vi "Begin.vi"(11 "Image Size":T1=enum."160x120") -> (0 "error out":errorcluster)   [LabVIEW 2013]
doc: "Called before other user functions, this VI is expected to open initial I/O refnums, load in file data, and do all program initialization. Notice that the <B>error out</B> terminal is simply used for data flow. Wiring it to other structures or subVIs ensures that this VI runs first."
uses:
  <vilib>/Rock Robotics/WPI/Camera/WPI_CameraImageSize.ctl
  <vilib>/Rock Robotics/SystemInterfaces/DIO/FPGA_DIOPWMChannel.ctl
  <vilib>/Rock Robotics/WPI/Camera/WPI_CameraWhite Balance Values.ctl
  <vilib>/Rock Robotics/WPI/Camera/WPI_CameraExposure Values.ctl
  <vilib>/Rock Robotics/WPI/Camera/WPI_CameraFrameRate.ctl
  <vilib>/Rock Robotics/WPI/DriverStation/WPI_DriverStationRobotMode2.ctl
  <vilib>/Rock Robotics/WPI/Joystick/WPI_JoystickDeviceEnum.ctl
  <vilib>/Rock Robotics/WPI/Solenoid/WPI_SolenoidChannel.ctl
  <vilib>/Rock Robotics/SystemInterfaces/DIO/FPGA_DIOChannel.ctl
  <vilib>/Rock Robotics/SystemInterfaces/DIO/FPGA_DIORelayChannel.ctl
  <vilib>/Rock Robotics/WPI/SafetyOutput/WPI_SafetyOutputConfigMenu.ctl
  <vilib>/Rock Robotics/SystemInterfaces/AI/FPGA_AIChannel.ctl
  <vilib>/Rock Robotics/SystemInterfaces/Typedef/FPGA_TypedefAnalogModule.ctl
  <vilib>/Rock Robotics/SystemInterfaces/AI/FPGA_AIGyroChannel.ctl
  <vilib>/Rock Robotics/SystemInterfaces/Typedef/FPGA_TypedefAnalogModuleForGyro.ctl
  <vilib>/Rock Robotics/SystemInterfaces/Typedef/FPGA_TypedefDigitalModule.ctl
  <vilib>/Rock Robotics/WPI/RobotDrive/WPI_RobotDriveOpen2MotorWithTalon.vi
  Robot Global Data.vi
  <vilib>/Rock Robotics/WPI/Solenoid/WPI_SolenoidOpenSingle.vi
  <vilib>/Rock Robotics/WPI/MotorControl/WPI_MotorControlOpen Victor.vi
  <vilib>/Rock Robotics/WPI/Counter/WPI_CounterDigitalInputToDigitalSource.vi
  <vilib>/Rock Robotics/WPI/Counter/WPI_CounterOpen Gear Tooth Sensor Mode.vi
  <vilib>/Rock Robotics/WPI/Compressor/WPI_CompressorGetSetRefNum.vi
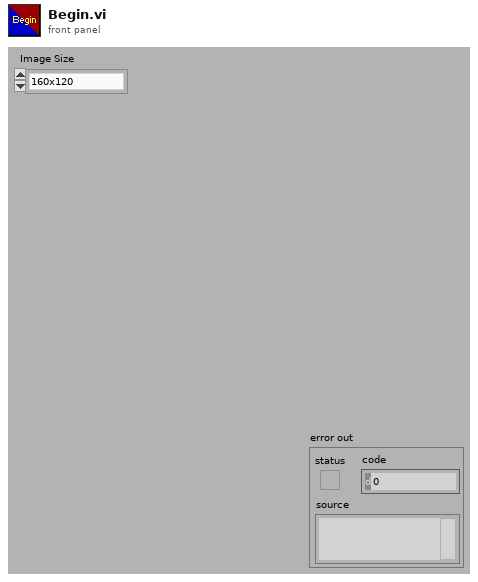
[diagram p1: front panel]
types:
  T1 = typedef "WPI_CameraImageSize.ctl" = enum16{"640x480", "320x240", "160x120"}
  T2 = typedef "WPI_SolenoidChannel.ctl" = enum8{"Solenoid 1", "Solenoid 2", "Solenoid 3", "Solenoid 4", "Solenoid 5", "Solenoid 6", "Solenoid 7", "Solenoid 8", "Invalid"}
  T3 = typedef "FPGA_TypedefDigitalModule.ctl" = enum16{"Digital Module 1", "Digital Module 2"}
  T4 = typedef "FPGA_DIOChannel.ctl" = enum8{"DIO 1", "DIO 2", "DIO 3", "DIO 4", "DIO 5", "DIO 6", "DIO 7", "DIO 8", "DIO 9", "DIO 10", "DIO 11", "DIO 12", "DIO 13", "DIO 14", "Invalid"}
  T5 = typedef "FPGA_TypedefAnalogModuleForGyro.ctl" = enum16{"Analog Module 1"}
  T6 = typedef "FPGA_AIGyroChannel.ctl" = enum8{"AI 1", "AI 2", "Invalid"}
  T7 = typedef "WPI_JoystickDeviceEnum.ctl" = enum16{"USB 1", "USB 2", "USB 3", "USB 4", "Kinect 1", "Kinect 2"}
  T8 = typedef "FPGA_TypedefAnalogModule.ctl" = enum16{"Analog Module 1", "Analog Module 2"}
  T9 = typedef "FPGA_AIChannel.ctl" = enum8{"AI 1", "AI 2", "AI 3", "AI 4", "AI 5", "AI 6", "AI 7", "AI 8", "Invalid"}
  T10 = typedef "WPI_SafetyOutputConfigMenu.ctl" = enum16{"Enable", "Disable"}
  T11 = typedef "FPGA_DIORelayChannel.ctl" = enum8{"Relay 1", "Relay 2", "Relay 3", "Relay 4", "Relay 5", "Relay 6", "Relay 7", "Relay 8", "Invalid"}
  T12 = typedef "FPGA_DIOPWMChannel.ctl" = enum8{"PWM 1", "PWM 2", "PWM 3", "PWM 4", "PWM 5", "PWM 6", "PWM 7", "PWM 8", "PWM 9", "PWM 10", "Invalid"}
  T13 = typedef "WPI_DriverStationRobotMode2.ctl" = enum16{"Autonomous Disabled", "Autonomous Enabled", "Teleop Disabled", "Teleop Enabled", "Timeout", "Finish", "Test Disabled", "Test Enabled"}
  T14 = typedef "WPI_CameraFrameRate.ctl" = u32
  T15 = typedef "WPI_CameraExposure Values.ctl" = enum16{"Auto", "Flicker-free 50 Hz", "Flicker-free 60 Hz", "Hold current"}
  T16 = typedef "WPI_CameraWhite Balance Values.ctl" = enum16{"Auto", "Fixed indoor", "Fixed outdoor 1", "Fixed outdoor 2", "Fixed fluorescent 1", "Fixed fluorescent 2", "Hold current"}
  T17 = typedef "WPI_SolenoidDevRef.ctl" = cluster{"DevStatus":errorcluster, "Solenoid Module":T18, "Forward Solenoid Channel":T2, "Reverse Solenoid Channel":T2}
  T18 = typedef "FPGA_TypedefSolenoidModule.ctl" = enum16{"Solenoid Module 1", "Solenoid Module 2"}
  T19 = typedef "WPI_JoystickDevRef.ctl" = cluster{"Device":T7}
  T20 = typedef "WPI_CameraDevRef.ctl" = cluster{"Camera Address":string, "CameraStatus":errorcluster, "Acquire Image Notifier":refnum<notifier>}
  T21 = typedef "WPI_CompressorDevRef.ctl" = cluster{"DevStatus":errorcluster, "DigitalInputDevRef":T22, "RelayDevRef":T23}
  T22 = typedef "WPI_DigitalInputDevRef.ctl" = cluster{"DevStatus":errorcluster, "DIO Channel":T4, "Digital Module":T3}
  T23 = typedef "WPI_RelayDevRef.ctl" = cluster{"DevStatus":errorcluster, "Relay Channel":T11, "Digital Module":T3, "Relay Direction":T24}
  T24 = typedef "WPI_RelayDirection.ctl" = enum16{"Both directions", "Forward only", "Reverse only"}
  T25 = typedef "WPI_RobotDriveDevRef.ctl" = cluster{"DevStatus":errorcluster, "Motors[]":T26[], "Square Inputs":bool, "Max Output":dbl, "Isochronous":bool}
  T26 = typedef "WPI_MotorControlDeviceRef.ctl" = cluster{"DeviceStatus":errorcluster, "Type":enum16{"PWM", "CAN"}, "PWM":cluster{"Digital Module":T3, "PWM Channel":T12, "DeadBand":T27}, "CAN":cluster{"Device Number":u8, "Control Mode":T28, "Semaphore":T29, "Max Vout":dbl}, "Invert":bool, "TransformRef":T30, "InvTransformRef":T30}
  T27 = typedef "WPI_PWMDeadband.ctl" = cluster{"Name":string, "maxPositivePwm":i32, "minPositivePwm":i32, "centerPwm":i32, "maxNegativePwm":i32, "minNegativePwm":i32, "angularRange":u16}
  T28 = typedef "WPI_CANJaguar_ControlMode.ctl" = enum8{"Percent VBus", "Current", "Speed", "Position", "Voltage"}
  T29 = typedef "Semaphore RefNum" = refnum<k1>
  T30 = typedef "WPI_PWMTransform_ConPane.ctl" = refnum<vi>
  T31 = typedef "WPI_ServoDeviceRef.ctl" = cluster{"DeviceStatus":errorcluster, "Digital Module":T3, "PWM Channel":T12, "DeadBand":T27}
  T32 = typedef "FPGA_CounterEncoderSourceConvertionLVSourceType.ctl" = cluster{"DevStatus":errorcluster, "AnalogTriggerMode?":bool, "DigitalMode":cluster{"Digital Module":T3, "DIO Channel":T33}, "AnalogTriggerMode":cluster{"AnalogTriggerIndex":T34, "OutputType":T35}}
  T33 = typedef "FPGA_DIODigitalSourceChannel.ctl" = enum8{"DIO 1", "DIO 2", "DIO 3", "DIO 4", "DIO 5", "DIO 6", "DIO 7", "DIO 8", "DIO 9", "DIO 10", "DIO 11", "DIO 12", "DIO 13", "DIO 14", "Disabled"}
  T34 = typedef "FPGA_AnalogTriggerIndex.ctl" = enum8{"Trig 0", "Trig 1", "Trig 2", "Trig 3", "Trig 4", "Trig 5", "Trig 6", "Trig 7", "Invalid"}
  T35 = typedef "FPGA_AnalogTriggerOutType.ctl" = enum16{"InWindow", "TriggerState", "Rising", "Falling"}
  T36 = typedef "WPI_EncoderDevRef.ctl" = cluster{"DevStatus":errorcluster, "EncoderIndex":T37, "CounterIndex":T38, "DistancePerCount":dbl, "Decoding Type":T39}
  T37 = typedef "FPGA_EncoderIdx.ctl" = enum8{"Enc 0", "Enc 1", "Enc 2", "Enc 3", "Invalid"}
  T38 = typedef "FPGA_CounterCtrSystemIndex.ctl" = enum8{"Ctr 0", "Ctr 1", "Ctr 2", "Ctr 3", "Ctr 4", "Ctr 5", "Ctr 6", "Ctr 7", "Invalid"}
  T39 = typedef "WPI_EncoderType.ctl" = enum16{"1x", "2x", "4x"}
  T40 = typedef "WPI_CounterDevRef.ctl" = cluster{"DevStatus":errorcluster, "CntIndex":T38}
  T41 = typedef "WPI_GyroDevRef.ctl" = cluster{"DevStatus":errorcluster, "Analog Module":T8, "Analog Channel":T9, "Offset":dbl, "Gain (VoltsPerDegree/Second)":dbl}
  T42 = typedef "WPI_AnalogChannelDevRef.ctl" = cluster{"DevStatus":errorcluster, "Analog Module":T8, "Analog Channel":T9}
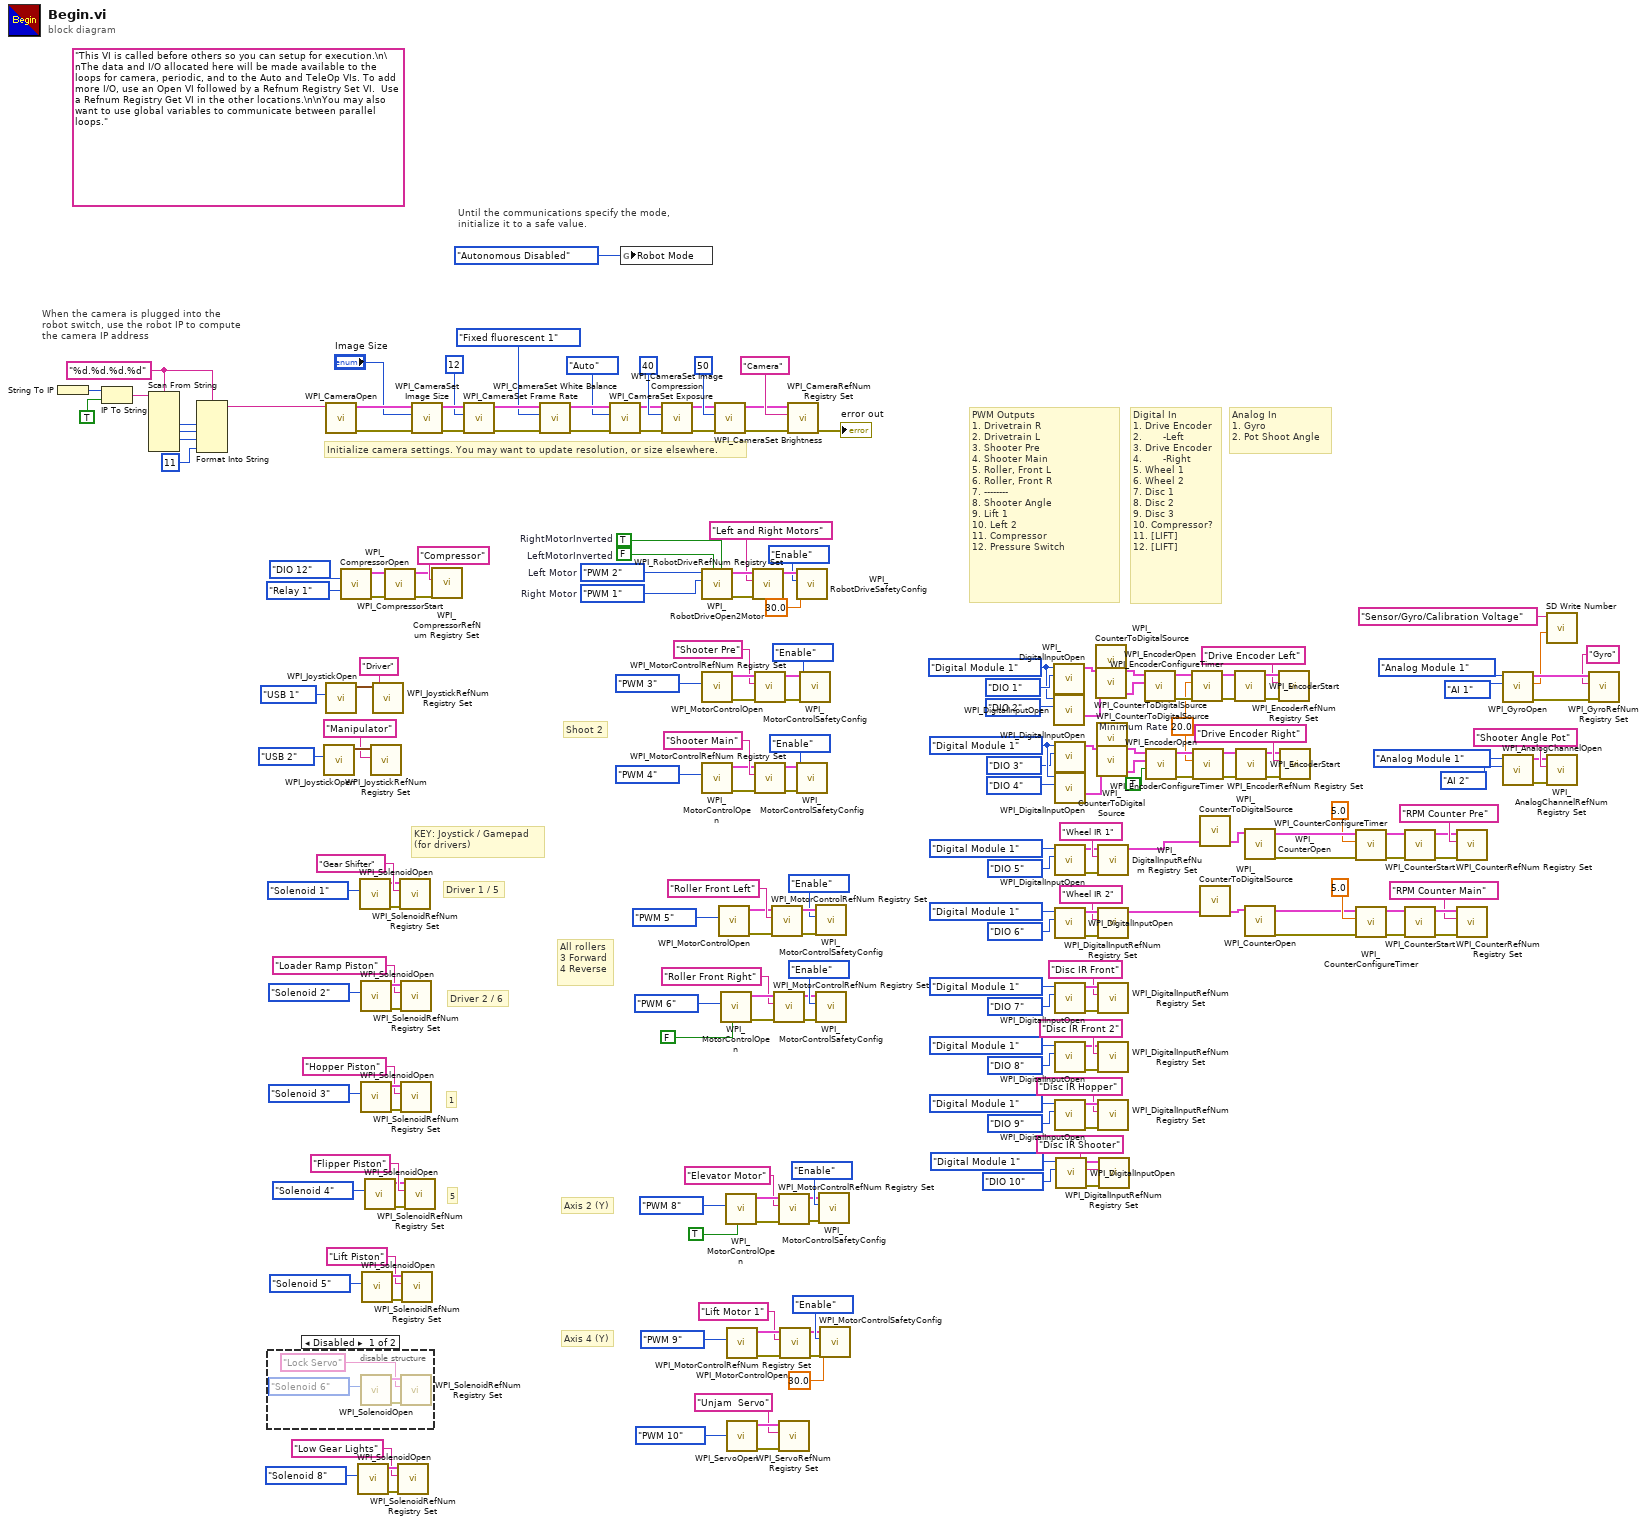
[diagram p0: block diagram]
diagram:
  w62 = 20.0  # Minimum Rate
  w101 = FPGA_TypedefDigitalModule."Digital Module 1" ("Digital Module (Module 1)")
  w108 = FPGA_TypedefDigitalModule."Digital Module 1" ("Digital Module (Module 1)")
  w187 = "%d.%d.%d.%d" ("format string")
  (unwired) "This VI is called before others so you can setup for execution.\n\nThe data and I/O allocated here will be made available to the loops for camera, periodic, and to the Auto and TeleOp VIs. To add more I/O, use an Open VI followed by a Refnum Registry Set VI.  Use a Refnum Registry Get VI in the other locations.\n\nYou may also want to use global variables to communicate between parallel loops."
  w36 = FPGA_DIOPWMChannel."PWM 1"  # Right Motor
  w37 = FPGA_DIOPWMChannel."PWM 2"  # Left Motor
  w219 = FALSE  # LeftMotorInverted
  w220 = TRUE  # RightMotorInverted
  # "KEY: Joystick / Gamepad\n(for drivers)"
  # "5"
  # "1"
  # "Axis 4 (Y)"
  # "Shoot 2"
  # "All rollers\n3 Forward\n4 Reverse"
  # "Axis 2 (Y)"
  # "Driver 2 / 6"
  # "Driver 1 / 5"
  # "Analog In\n1. Gyro\n2. Pot Shoot Angle"
  # "Digital In\n1. Drive Encoder\n2.       -Left\n3. Drive Encoder\n4.       -Right\n5. Wheel 1\n6. Wheel 2\n7. Disc 1\n8. Disc 2\n9. Disc 3\n10. Compressor?\n11. [LIFT]\n12. [LIFT]"
  # "PWM Outputs\n1. Drivetrain R\n2. Drivetrain L\n3. Shooter Pre\n4. Shooter Main\n5. Roller, Front L\n6. Roller, Front R\n7. --------\n8. Shooter Angle\n9. Lift 1\n10. Left 2\n11. Compressor\n12. Pressure Switch"
  # "Until the communications specify the mode,\ninitialize it to a safe value."
  # "When the camera is plugged into the\nrobot switch, use the robot IP to compute\nthe camera IP address"
  # "Initialize camera settings. You may want to update resolution, or size elsewhere."
  n1 = String To IP() -> (0:w194:u32)  [unwired: 1 in]
  n2 = IP To String(1:TRUE ("dot notation? (F)"), 2:w194) -> (0:w192:string)
  n3 = Scan From String(format string=w187, input string=w192) -> (output 1=w191:i32, output 2=w190:i32, output 3=w189:i32)  [unwired: 7 in, 3 out]
  n4 = Format Into String(format string=w187, w191, w190, w189, 11 ("Compression")) -> (resulting string=w183:string)  [unwired: 2 in, 1 out]
  n5 = disable-structure shown="Disabled" {
    frame Disabled {
      n6 = call-poly <vilib>:"WPI_SolenoidOpen.vi"("Solenoid Channel"=WPI_SolenoidChannel."Solenoid 6") -> ("error out"=w223:errorcluster, "SolenoidDevRef"=w224:T17)  [unwired: 9 in]
      n7 = call <vilib>:"WPI_SolenoidRefNum Registry Set.vi"("error in (no error)"=w223, "refnum name"="Lock Servo", "SolenoidDevRef"=w224) -> ()  [unwired: 7 in, 2 out]
    }
    frame Enabled {
    }
  }
  n8 = call <vilib>:"WPI_JoystickOpen.vi"("JoystickDevice"=WPI_JoystickDeviceEnum."USB 2") -> ("JoystickDevRef"=w64:T19)  [unwired: 10 in]
  n9 = call <vilib>:"WPI_CameraOpen.vi"("Camera Address"=w183) -> ("error out"=w206:errorcluster, "CameraDevRef"=w207:T20)  [unwired: 1 in, 8 out]
  n10 = call <vilib>:"WPI_JoystickOpen.vi"("JoystickDevice"=WPI_JoystickDeviceEnum."USB 1") -> ("JoystickDevRef"=w181:T19)  [unwired: 10 in]
  n11 = call <vilib>:"WPI_CompressorOpen.vi"("Pressure Switch DIO Channel"=FPGA_DIOChannel."DIO 12", "Relay Channel"=FPGA_DIORelayChannel."Relay 1") -> ("CompressorDevRef"=w35:T21, "error out"=w34:errorcluster)  [unwired: 12 in]
  n12 = call-poly <vilib>:"WPI_SolenoidOpen.vi"("Solenoid Channel"=WPI_SolenoidChannel."Solenoid 8") -> ("error out"=w5:errorcluster, "SolenoidDevRef"=w4:T17)  [unwired: 9 in]
  n13 = call-poly <vilib>:"WPI_SolenoidOpen.vi"("Solenoid Channel"=WPI_SolenoidChannel."Solenoid 1") -> ("error out"=w59:errorcluster, "SolenoidDevRef"=w60:T17)  [unwired: 9 in]
  n14 = call-poly <vilib>:"WPI_SolenoidOpen.vi"("Solenoid Channel"=WPI_SolenoidChannel."Solenoid 2") -> ("error out"=w177:errorcluster, "SolenoidDevRef"=w176:T17)  [unwired: 9 in]
  n15 = call-poly <vilib>:"WPI_SolenoidOpen.vi"("Solenoid Channel"=WPI_SolenoidChannel."Solenoid 3") -> ("error out"=w173:errorcluster, "SolenoidDevRef"=w172:T17)  [unwired: 9 in]
  n16 = call-poly <vilib>:"WPI_SolenoidOpen.vi"("Solenoid Channel"=WPI_SolenoidChannel."Solenoid 5") -> ("error out"=w52:errorcluster, "SolenoidDevRef"=w51:T17)  [unwired: 9 in]
  n17 = call-poly <vilib>:"WPI_SolenoidOpen.vi"("Solenoid Channel"=WPI_SolenoidChannel."Solenoid 4") -> ("error out"=w55:errorcluster, "SolenoidDevRef"=w56:T17)  [unwired: 9 in]
  n18 = call <vilib>:"WPI_JoystickRefNum Registry Set.vi"("refnum name"="Manipulator", "JoystickDevRef"=w64) -> ()  [unwired: 8 in, 2 out]
  n19 = call <vilib>:"WPI_JoystickRefNum Registry Set.vi"("refnum name"="Driver", "JoystickDevRef"=w181) -> ()  [unwired: 8 in, 2 out]
  n20 = call <vilib>:"WPI_CompressorStart.vi"("error in (no error)"=w34, "CompressorDevRef"=w35) -> ("error out"=w32:errorcluster, "CompressorDevRef"=w33:T21)  [unwired: 8 in]
  n21 = call <vilib>:"WPI_SolenoidRefNum Registry Set.vi"("error in (no error)"=w5, "refnum name"="Low Gear Lights", "SolenoidDevRef"=w4) -> ()  [unwired: 7 in, 2 out]
  n22 = call <vilib>:"WPI_SolenoidRefNum Registry Set.vi"("error in (no error)"=w59, "refnum name"="Gear Shifter", "SolenoidDevRef"=w60) -> ()  [unwired: 7 in, 2 out]
  n23 = call <vilib>:"WPI_SolenoidRefNum Registry Set.vi"("error in (no error)"=w177, "refnum name"="Loader Ramp Piston", "SolenoidDevRef"=w176) -> ()  [unwired: 7 in, 2 out]
  n24 = call <vilib>:"WPI_SolenoidRefNum Registry Set.vi"("error in (no error)"=w173, "refnum name"="Hopper Piston", "SolenoidDevRef"=w172) -> ()  [unwired: 7 in, 2 out]
  n25 = call <vilib>:"WPI_SolenoidRefNum Registry Set.vi"("error in (no error)"=w52, "refnum name"="Lift Piston", "SolenoidDevRef"=w51) -> ()  [unwired: 7 in, 2 out]
  n26 = call <vilib>:"WPI_SolenoidRefNum Registry Set.vi"("error in (no error)"=w55, "refnum name"="Flipper Piston", "SolenoidDevRef"=w56) -> ()  [unwired: 7 in, 2 out]
  n27 = call <vilib>:"WPI_CameraSet Image Size.vi"("error in (no error)"=w206, "Image Size"="Image Size", "CameraDevRef"=w207) -> ("error out"=w205:errorcluster, "CameraDevRef Out"=w208:T20)  [unwired: 7 out]
  n28 = call <vilib>:"WPI_CompressorRefNum Registry Set.vi"("error in (no error)"=w32, "refnum name"="Compressor", "CompressorDevRef"=w33) -> ()  [unwired: 7 in, 2 out]
  n29 = call <vilib>:"WPI_CameraSet Frame Rate.vi"("error in (no error)"=w205, "Frame Rate (fps)"=T14 12, "CameraDevRef"=w208) -> ("error out"=w204:errorcluster, "CameraDevRef Out"=w210:T20)  [unwired: 7 out]
  n30 = call <vilib>:"WPI_CameraSet White Balance.vi"("error in (no error)"=w204, "White Balance"=WPI_CameraWhite_Balance_Values."Fixed fluorescent 1", "CameraDevRef"=w210) -> ("error out"=w203:errorcluster, "CameraDevRef Out"=w209:T20)  [unwired: 7 out]
  n31 = call <vilib>:"WPI_CameraSet Exposure.vi"("error in (no error)"=w203, "Exposure"=WPI_CameraExposure_Values."Auto", "CameraDevRef"=w209) -> ("error out"=w202:errorcluster, "CameraDevRef Out"=w212:T20)  [unwired: 7 out]
  n32 = global write "Robot Global Data.vi" "Robot Mode"(WPI_DriverStationRobotMode2."Autonomous Disabled" ("Robot Mode")) -> ()
  n33 = call <vilib>:"WPI_CameraSet Image Compression.vi"("error in (no error)"=w202, "Compression"=40, "CameraDevRef"=w212) -> ("error out"=w201:errorcluster, "CameraDevRef Out"=w211:T20)  [unwired: 7 out]
  n34 = call-poly <vilib>:"WPI_RobotDriveOpen2Motor.vi"("Right Motor Inverted"=w220, "Left Motor Inverted"=w219, "Right Motor"=w36, "Left Motor"=w37) -> ("error out"=w215:errorcluster, "RobotDriveDevRef"=w217:T25)  [unwired: 1 in, 5 out]
  n35 = call-poly <vilib>:"WPI_MotorControlOpen.vi"("PWM Channel"=FPGA_DIOPWMChannel."PWM 3") -> ("error out"=w142:errorcluster, "MotorControlDeviceRef"=w141:T26)  [unwired: 9 in]
  n36 = call-poly <vilib>:"WPI_MotorControlOpen.vi"("PWM Channel"=FPGA_DIOPWMChannel."PWM 4") -> ("error out"=w143:errorcluster, "MotorControlDeviceRef"=w144:T26)  [unwired: 9 in]
  n37 = call <vilib>:"WPI_CameraSet Brightness.vi"("error in (no error)"=w201, "Brightness"=50, "CameraDevRef"=w211) -> ("error out"=w199:errorcluster, "CameraDevRef Out"=w200:T20)  [unwired: 7 out]
  n38 = call-poly <vilib>:"WPI_MotorControlOpen.vi"("PWM Channel"=FPGA_DIOPWMChannel."PWM 5") -> ("error out"=w151:errorcluster, "MotorControlDeviceRef"=w152:T26)  [unwired: 9 in]
  n39 = call-poly <vilib>:"WPI_MotorControlOpen.vi"("Invert"=FALSE, "PWM Channel"=FPGA_DIOPWMChannel."PWM 6") -> ("error out"=w150:errorcluster, "MotorControlDeviceRef"=w149:T26)  [unwired: 8 in]
  n40 = call-poly <vilib>:"WPI_MotorControlOpen.vi"("Invert"=TRUE, "PWM Channel"=FPGA_DIOPWMChannel."PWM 8") -> ("error out"=w170:errorcluster, "MotorControlDeviceRef"=w169:T26)  [unwired: 8 in]
  n41 = call-poly <vilib>:"WPI_MotorControlOpen.vi"("PWM Channel"=FPGA_DIOPWMChannel."PWM 9") -> ("error out"=w166:errorcluster, "MotorControlDeviceRef"=w165:T26)  [unwired: 9 in]
  n42 = call <vilib>:"WPI_ServoOpen.vi"("PWM Channel"=FPGA_DIOPWMChannel."PWM 10") -> ("error out"=w9:errorcluster, "ServoDeviceRef"=w8:T31)  [unwired: 9 in]
  n43 = call <vilib>:"WPI_RobotDriveRefNum Registry Set.vi"("error in (no error)"=w215, "refnum name"="Left and Right Motors", "RobotDriveDevRef"=w217) -> ("RobotDriveDevRef"=w186:T25)  [unwired: 8 out]
  n44 = call <vilib>:"WPI_MotorControlRefNum Registry Set.vi"("error in (no error)"=w142, "refnum name"="Shooter Pre", "MotorControlDevRef"=w141) -> ("error out"=w136:errorcluster, "MotorControlDevRef"=w135:T26)  [unwired: 7 in]
  n45 = call <vilib>:"WPI_MotorControlRefNum Registry Set.vi"("error in (no error)"=w143, "refnum name"="Shooter Main", "MotorControlDevRef"=w144) -> ("error out"=w131:errorcluster, "MotorControlDevRef"=w132:T26)  [unwired: 7 in]
  n46 = call <vilib>:"WPI_MotorControlRefNum Registry Set.vi"("error in (no error)"=w151, "refnum name"="Roller Front Left", "MotorControlDevRef"=w152) -> ("error out"=w129:errorcluster, "MotorControlDevRef"=w130:T26)  [unwired: 7 in]
  n47 = call <vilib>:"WPI_MotorControlRefNum Registry Set.vi"("error in (no error)"=w150, "refnum name"="Roller Front Right", "MotorControlDevRef"=w149) -> ("error out"=w126:errorcluster, "MotorControlDevRef"=w125:T26)  [unwired: 7 in]
  n48 = call <vilib>:"WPI_MotorControlRefNum Registry Set.vi"("error in (no error)"=w170, "refnum name"="Elevator Motor", "MotorControlDevRef"=w169) -> ("error out"=w123:errorcluster, "MotorControlDevRef"=w122:T26)  [unwired: 7 in]
  n49 = call <vilib>:"WPI_ServoRefNum Registry Set.vi"("error in (no error)"=w9, "refnum name"="Unjam  Servo", "ServoDeviceRef"=w8) -> ()  [unwired: 7 in, 2 out]
  n50 = call <vilib>:"WPI_MotorControlRefNum Registry Set.vi"("error in (no error)"=w166, "refnum name"="Lift Motor 1", "MotorControlDevRef"=w165) -> ("error out"=w120:errorcluster, "MotorControlDevRef"=w119:T26)  [unwired: 7 in]
  n51 = call <vilib>:"WPI_CameraRefNum Registry Set.vi"("error in (no error)"=w199, "refnum name"="Camera", "CameraDevRef"=w200) -> ("error out"=→"error out":errorcluster)  [unwired: 8 out]
  n52 = call <vilib>:"WPI_RobotDriveSafetyConfig.vi"("timeout (s)"=30.0, "mode"=WPI_SafetyOutputConfigMenu."Enable", "RobotDriveDevRef"=w186) -> ()  [unwired: 7 in, 2 out]
  n53 = call <vilib>:"WPI_MotorControlSafetyConfig.vi"("error in (no error)"=w131, "mode"=WPI_SafetyOutputConfigMenu."Enable", "MotorControlDevRef"=w132) -> ()  [unwired: 7 in, 2 out]
  n54 = call <vilib>:"WPI_MotorControlSafetyConfig.vi"("error in (no error)"=w136, "mode"=WPI_SafetyOutputConfigMenu."Enable", "MotorControlDevRef"=w135) -> ()  [unwired: 7 in, 2 out]
  n55 = call <vilib>:"WPI_MotorControlSafetyConfig.vi"("error in (no error)"=w129, "mode"=WPI_SafetyOutputConfigMenu."Enable", "MotorControlDevRef"=w130) -> ()  [unwired: 7 in, 2 out]
  n56 = call <vilib>:"WPI_MotorControlSafetyConfig.vi"("error in (no error)"=w126, "mode"=WPI_SafetyOutputConfigMenu."Enable", "MotorControlDevRef"=w125) -> ()  [unwired: 7 in, 2 out]
  n57 = call <vilib>:"WPI_MotorControlSafetyConfig.vi"("error in (no error)"=w123, "mode"=WPI_SafetyOutputConfigMenu."Enable", "MotorControlDevRef"=w122) -> ()  [unwired: 7 in, 2 out]
  n58 = call <vilib>:"WPI_MotorControlSafetyConfig.vi"("error in (no error)"=w120, "timeout (s)"=30.0, "mode"=WPI_SafetyOutputConfigMenu."Enable", "MotorControlDevRef"=w119) -> ()  [unwired: 6 in, 2 out]
  n59 = call <vilib>:"WPI_DigitalInputOpen.vi"("DIO Channel"=FPGA_DIOChannel."DIO 1", "Digital Module (Module 1)"=w108) -> ("DigitalInputDevRef"=w109:T22)  [unwired: 8 in, 1 out]
  n60 = call <vilib>:"WPI_DigitalInputOpen.vi"("DIO Channel"=FPGA_DIOChannel."DIO 2", "Digital Module (Module 1)"=w108) -> ("DigitalInputDevRef"=w112:T22)  [unwired: 8 in, 1 out]
  n61 = call <vilib>:"WPI_DigitalInputOpen.vi"("DIO Channel"=FPGA_DIOChannel."DIO 3", "Digital Module (Module 1)"=w101) -> ("DigitalInputDevRef"=w100:T22)  [unwired: 8 in, 1 out]
  n62 = call <vilib>:"WPI_DigitalInputOpen.vi"("DIO Channel"=FPGA_DIOChannel."DIO 4", "Digital Module (Module 1)"=w101) -> ("DigitalInputDevRef"=w97:T22)  [unwired: 8 in, 1 out]
  n63 = call <vilib>:"WPI_DigitalInputOpen.vi"("DIO Channel"=FPGA_DIOChannel."DIO 5", "Digital Module (Module 1)"=FPGA_TypedefDigitalModule."Digital Module 1") -> ("error out"=w157:errorcluster, "DigitalInputDevRef"=w158:T22)  [unwired: 8 in]
  n64 = call <vilib>:"WPI_DigitalInputOpen.vi"("DIO Channel"=FPGA_DIOChannel."DIO 6", "Digital Module (Module 1)"=FPGA_TypedefDigitalModule."Digital Module 1") -> ("error out"=w88:errorcluster, "DigitalInputDevRef"=w87:T22)  [unwired: 8 in]
  n65 = call <vilib>:"WPI_DigitalInputOpen.vi"("DIO Channel"=FPGA_DIOChannel."DIO 7", "Digital Module (Module 1)"=FPGA_TypedefDigitalModule."Digital Module 1") -> ("error out"=w84:errorcluster, "DigitalInputDevRef"=w85:T22)  [unwired: 8 in]
  n66 = call <vilib>:"WPI_DigitalInputOpen.vi"("DIO Channel"=FPGA_DIOChannel."DIO 8", "Digital Module (Module 1)"=FPGA_TypedefDigitalModule."Digital Module 1") -> ("error out"=w77:errorcluster, "DigitalInputDevRef"=w76:T22)  [unwired: 8 in]
  n67 = call <vilib>:"WPI_DigitalInputOpen.vi"("DIO Channel"=FPGA_DIOChannel."DIO 9", "Digital Module (Module 1)"=FPGA_TypedefDigitalModule."Digital Module 1") -> ("error out"=w74:errorcluster, "DigitalInputDevRef"=w75:T22)  [unwired: 8 in]
  n68 = call <vilib>:"WPI_DigitalInputOpen.vi"("DIO Channel"=FPGA_DIOChannel."DIO 10", "Digital Module (Module 1)"=FPGA_TypedefDigitalModule."Digital Module 1") -> ("error out"=w40:errorcluster, "DigitalInputDevRef"=w39:T22)  [unwired: 8 in]
  n69 = call-poly <vilib>:"WPI_CounterToDigitalSource.vi"("DigitalInputDevRef"=w109) -> ("Digital Source"=w110:T32)  [unwired: 6 in]
  n70 = call-poly <vilib>:"WPI_CounterToDigitalSource.vi"("DigitalInputDevRef"=w112) -> ("Digital Source"=w111:T32)  [unwired: 6 in]
  n71 = call-poly <vilib>:"WPI_CounterToDigitalSource.vi"("DigitalInputDevRef"=w100) -> ("Digital Source"=w99:T32)  [unwired: 6 in]
  n72 = call-poly <vilib>:"WPI_CounterToDigitalSource.vi"("DigitalInputDevRef"=w97) -> ("Digital Source"=w98:T32)  [unwired: 6 in]
  n73 = call <vilib>:"WPI_DigitalInputRefNum Registry Set.vi"("error in (no error)"=w157, "refnum name"="Wheel IR 1", "DigitalInputDevRef"=w158) -> ("DigitalInputDevRef"=w30:T22)  [unwired: 7 in, 1 out]
  n74 = call <vilib>:"WPI_DigitalInputRefNum Registry Set.vi"("error in (no error)"=w88, "refnum name"="Wheel IR 2", "DigitalInputDevRef"=w87) -> ("DigitalInputDevRef"=w12:T22)  [unwired: 7 in, 1 out]
  n75 = call <vilib>:"WPI_DigitalInputRefNum Registry Set.vi"("error in (no error)"=w84, "refnum name"="Disc IR Front", "DigitalInputDevRef"=w85) -> ()  [unwired: 7 in, 2 out]
  n76 = call <vilib>:"WPI_DigitalInputRefNum Registry Set.vi"("error in (no error)"=w77, "refnum name"="Disc IR Front 2", "DigitalInputDevRef"=w76) -> ()  [unwired: 7 in, 2 out]
  n77 = call <vilib>:"WPI_DigitalInputRefNum Registry Set.vi"("error in (no error)"=w74, "refnum name"="Disc IR Hopper", "DigitalInputDevRef"=w75) -> ()  [unwired: 7 in, 2 out]
  n78 = call <vilib>:"WPI_DigitalInputRefNum Registry Set.vi"("error in (no error)"=w40, "refnum name"="Disc IR Shooter", "DigitalInputDevRef"=w39) -> ()  [unwired: 7 in, 2 out]
  n79 = call <vilib>:"WPI_EncoderOpen.vi"("BSource"=w111, "ASource"=w110) -> ("error out"=w116:errorcluster, "EncoderDevRef"=w115:T36)  [unwired: 8 in]
  n80 = call <vilib>:"WPI_EncoderOpen.vi"("Invert Direction (False)"=TRUE, "BSource"=w98, "ASource"=w99) -> ("error out"=w93:errorcluster, "EncoderDevRef"=w94:T36)  [unwired: 7 in]
  n81 = call <vilib>:"WPI_EncoderConfigureTimer.vi"("error in (no error)"=w116, "Minimum Rate"=w62, "EncoderDevRef"=w115) -> ("error out"=w114:errorcluster, "EncoderDevRef"=w113:T36)  [unwired: 7 in]
  n82 = call <vilib>:"WPI_EncoderConfigureTimer.vi"("error in (no error)"=w93, "Minimum Rate"=w62, "EncoderDevRef"=w94) -> ("error out"=w95:errorcluster, "EncoderDevRef"=w96:T36)  [unwired: 7 in]
  n83 = call-poly <vilib>:"WPI_CounterToDigitalSource.vi"("DigitalInputDevRef"=w30) -> ("Digital Source"=w31:T32)  [unwired: 6 in]
  n84 = call-poly <vilib>:"WPI_CounterToDigitalSource.vi"("DigitalInputDevRef"=w12) -> ("Digital Source"=w13:T32)  [unwired: 6 in]
  n85 = call <vilib>:"WPI_EncoderStart.vi"("error in (no error)"=w114, "EncoderDevRef"=w113) -> ("error out"=w107:errorcluster, "EncoderDevRef"=w106:T36)  [unwired: 8 in]
  n86 = call <vilib>:"WPI_EncoderStart.vi"("error in (no error)"=w95, "EncoderDevRef"=w96) -> ("error out"=w102:errorcluster, "EncoderDevRef"=w103:T36)  [unwired: 8 in]
  n87 = call-poly <vilib>:"WPI_CounterOpen.vi"("Source"=w31) -> ("error out"=w28:errorcluster, "CounterDevRef"=w29:T40)  [unwired: 9 in]
  n88 = call-poly <vilib>:"WPI_CounterOpen.vi"("Source"=w13) -> ("error out"=w15:errorcluster, "CounterDevRef"=w14:T40)  [unwired: 9 in]
  n89 = call <vilib>:"WPI_EncoderRefNum Registry Set.vi"("error in (no error)"=w107, "refnum name"="Drive Encoder Left", "EncoderDevRef"=w106) -> ()  [unwired: 7 in, 2 out]
  n90 = call <vilib>:"WPI_EncoderRefNum Registry Set.vi"("error in (no error)"=w102, "refnum name"="Drive Encoder Right", "EncoderDevRef"=w103) -> ()  [unwired: 7 in, 2 out]
  n91 = call <vilib>:"WPI_CounterConfigureTimer.vi"("error in (no error)"=w28, "MaxPeriod (sec)"=5.0, "CounterDevRef in"=w29) -> ("error out"=w26:errorcluster, "CounterDevRef out"=w25:T40)  [unwired: 7 in]
  n92 = call <vilib>:"WPI_CounterConfigureTimer.vi"("error in (no error)"=w15, "MaxPeriod (sec)"=5.0, "CounterDevRef in"=w14) -> ("error out"=w17:errorcluster, "CounterDevRef out"=w18:T40)  [unwired: 7 in]
  n93 = call <vilib>:"WPI_CounterStart.vi"("error in (no error)"=w26, "CounterDevRef in"=w25) -> ("error out"=w24:errorcluster, "CounterDevRef out"=w23:T40)  [unwired: 8 in]
  n94 = call <vilib>:"WPI_CounterStart.vi"("error in (no error)"=w17, "CounterDevRef in"=w18) -> ("error out"=w19:errorcluster, "CounterDevRef out"=w20:T40)  [unwired: 8 in]
  n95 = call <vilib>:"WPI_CounterRefNum Registry Set.vi"("error in (no error)"=w24, "refnum name"="RPM Counter Pre", "CounterDevRef"=w23) -> ()  [unwired: 7 in, 2 out]
  n96 = call <vilib>:"WPI_CounterRefNum Registry Set.vi"("error in (no error)"=w19, "refnum name"="RPM Counter Main", "CounterDevRef"=w20) -> ()  [unwired: 7 in, 2 out]
  n97 = call <vilib>:"WPI_GyroOpen.vi"("Analog Channel"=FPGA_AIGyroChannel."AI 1", "Analog Module (Module 1)"=FPGA_TypedefAnalogModuleForGyro."Analog Module 1") -> ("error out"=w162:errorcluster, "Calibrated Center Voltage Out"=w45:dbl, "GyroDevRef"=w161:T41)  [unwired: 7 in]
  n98 = call <vilib>:"WPI_AnalogChannelOpen.vi"("Analog Channel"=FPGA_AIChannel."AI 2", "Analog Module (Module 1)"=FPGA_TypedefAnalogModule."Analog Module 1") -> ("error out"=w68:errorcluster, "AIDeviceRef"=w69:T42)  [unwired: 8 in]
  n99 = call <vilib>:"SD Write Number.vi"("Numeric"=w45, "Name"="Sensor/Gyro/Calibration Voltage") -> ()  [unwired: 8 in, 2 out]
  n100 = call <vilib>:"WPI_AnalogChannelRefNum Registry Set.vi"("error in (no error)"=w68, "refnum name"="Shooter Angle Pot", "AIDeviceRef"=w69) -> ()  [unwired: 7 in, 2 out]
  n101 = call <vilib>:"WPI_GyroRefNum Registry Set.vi"("error in (no error)"=w162, "refnum name"="Gyro", "GyroDevRef"=w161) -> ()  [unwired: 7 in, 2 out]
